vi "Handle Chart Menu Activation.vi"(7 "Channel Names":string[](array[string]), 9 "Coords":T1, 10 "MenuRef":refnum<k9>, 11 "CtlRef":refnum<vi>) -> (1 "Channel Index":i32)   [LabVIEW 2018, in "Visualization.lvlib" / "VisualizeBase.lvclass"]
uses:
  VisualizeBase/VisualizeBase_class/VisualizeBase.lvclass
  <vilib>/Utility/miscctls.llb/LVPoint32TypeDef.ctl
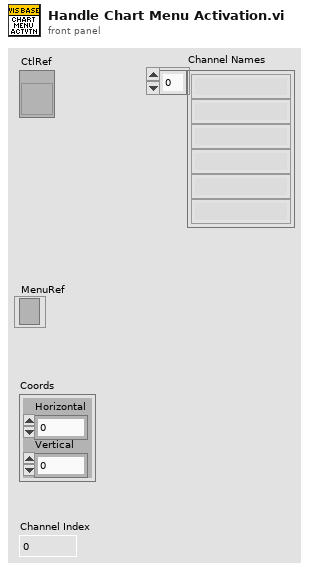
[diagram p1: front panel]
types:
  T1 = typedef "LVPoint32TypeDef.ctl" = cluster{"Horizontal":i32, "Vertical":i32}
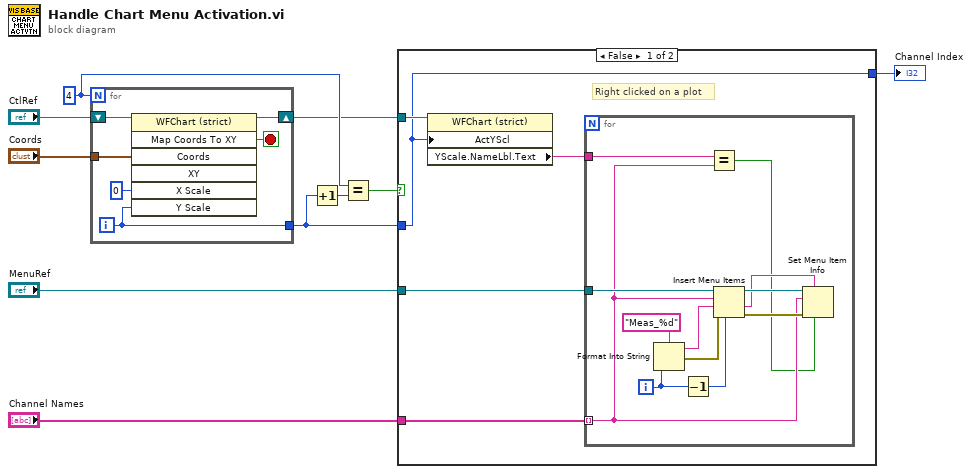
[diagram p0: block diagram]
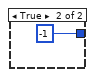
[diagram p2: hidden frame]
diagram:
  w9 = 4
  n1 = for {
    N: w9 -> [_]
    tunnel: "Coords" -> [w15]
    tunnel: [w12] -> w7
    shift-right: [w11] -> w6
    shift-left: "CtlRef" -> [w16]
    i -> [w12]
    stop <- w13 stop-if-true
    n2 = invoke class="WFChart (strict)" method="Map Coords To XY"(reference=w16, "Coords"=w15, "X Scale"=0, "Y Scale"=w12) -> (reference out=w11:refnum<vi>, "Map Coords To XY"=w13:bool)  [unwired: 3 in, 5 out]
  }
  n3 = Increment(x=w7) -> (x+1=w10:i32)
  n4 = Equal?(x=w9, y=w10) -> (x = y?=w8:bool)
  n5 = case shown="False" w8 {
    tunnel: "MenuRef" -> [w21 _]
    tunnel: w7 -> [w17 _]
    tunnel: w6 -> [w20 _]
    tunnel: "Channel Names" -> [w18 _]
    tunnel: [w17 -1] -> w1
    frame False {
      # "Right clicked on a plot"
      n6 = property class="WFChart (strict)"(reference=w20, "ActYScl"=w17) -> ("YScale.NameLbl.Text"=w19:string)  [unwired: 1 in, 2 out]
      n7 = for {
        tunnel: w21 -> [w33]
        tunnel: w18 -> [w26] mode=indexing
        tunnel: w19 -> [w29]
        i -> [w30]
        n8 = Format Into String(format string="Meas_%d", w30) -> (resulting string=w32:string, error out=w23:errorcluster)  [unwired: 2 in]
        n9 = Decrement(x=w30) -> (x-1=w31:i32)
        n10 = Equal?(x=w29, y=w26) -> (x = y?=w24:bool)
        n11 = Insert Menu Items(4:w31, 6:w23, 7:w32, 8:w26, 9:w33) -> (0:w28:errorcluster, 1:w25:string, 3:w27:refnum<k9>)  [unwired: 1 in]
        n12 = Set Menu Item Info(6:w24, 7:w25, 8:w28, 10:w26, 11:w27) -> ()  [unwired: 2 in, 2 out]
      }
    }
    frame True {
    }
  }
  "Channel Index" <- w1
